vi "displayDate.vi"(8 "error in (no error)":errorcluster, 10 "MonthDisplay":refnum<class "DateUserInterface.lvclass">, 11 "WhichMonth in":refnum<class "WhichMonth.lvclass">) -> (0 "error out":errorcluster, 3 "WhichMonth out":refnum<class "WhichMonth.lvclass">)   [LabVIEW 2018, in "WhichMonth.lvclass"]
uses:
  WhichMonth.lvclass
  MonthDisplay/DateUserInterface.lvclass
  WhichMonth.lvclass/WhichMonth.ctl
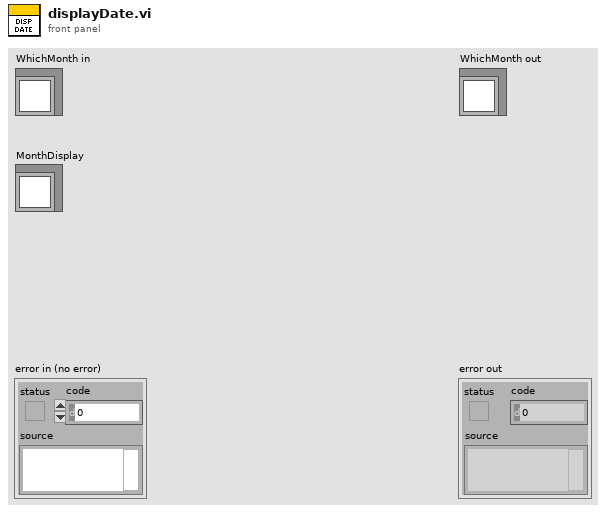
[diagram p1: front panel]
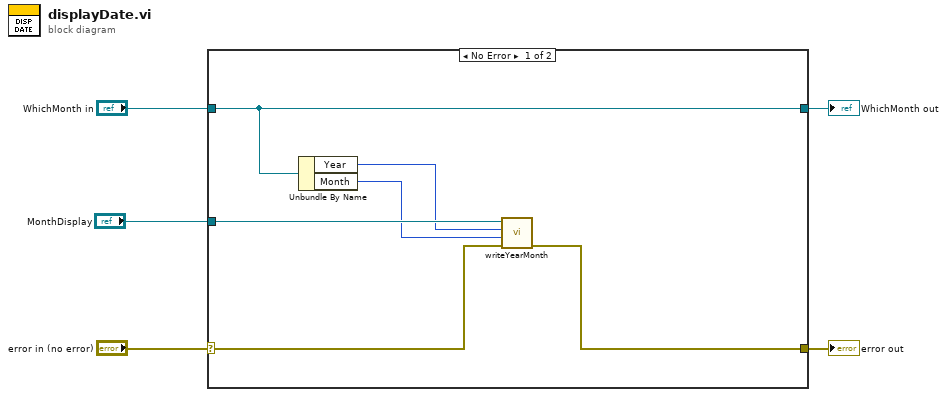
[diagram p0: block diagram]
diagram:
  n1 = case shown="No Error" "error in (no error)" {
    selector: "error in (no error)" -> [w9 w13]
    tunnel: [w8 w13] -> w4
    tunnel: [w11 w12] -> w2
    tunnel: "WhichMonth in" -> [w11 w12]
    tunnel: "MonthDisplay" -> [w10 _]
    frame No Error {
      n2 = Unbundle By Name(w11) -> ("Year"=w7:i32, "Month"=w6:i32)
      n3 = call "writeYearMonth.vi"("error in (no error)"=w9, "Month"=w6, "Year"=w7, "MonthDisplay in"=w10) -> ("error out"=w8:errorcluster)  [unwired: 6 in, 1 out]
    }
    frame Error {
    }
  }
  "error out" <- w4
  "WhichMonth out" <- w2
